vi "Chat Message Callback.vi"(7 "Owner":refnum<class>, 11 "Message":refnum<class "Message.lvclass">) -> (0 "error out":errorcluster)   [LabVIEW 2020, in "LV Chat Server.lvclass"]
uses:
  LV Chat Server.lvclass
  <vilib>/IlluminatedG/lv-msg-simple/Stream-Simple-Msg/Message/Message.lvclass
  LV Chat Server.lvclass/LV Chat Server.ctl
  Data Types/Message.ctl
  Data Types/Message ID.ctl
  9b2631c7-d2a0-400d-8d9b-28026d0b08d4.vi
  8fd8f42d-e5b1-4272-a4de-ff1efb915e34.vi
  a0ad2d85-71bd-4b38-8ce3-2817e254df22.vi
  a0ad2d85-71bd-4b38-8ce3-2817e254df22.vi/43e93f4b-eb60-4448-b7e4-56a49cc750fb.vi
  a0ad2d85-71bd-4b38-8ce3-2817e254df22.vi/43e93f4b-eb60-4448-b7e4-56a49cc750fb.vi/4b61994f-5270-44fc-a580-5e93e6c23fba.vi
  <vilib>/IlluminatedG/lv-stream/stream/Write Formatted Data.vi
  <vilib>/IlluminatedG/lv-msg-simple/Stream-Simple-Msg/Message/Data and Type.vi
  <vilib>/IlluminatedG/lv-msg-simple/Stream-Simple-Msg/Manager/Get Endpoints.vi
  <vilib>/IlluminatedG/lv-msg-simple/Stream-Simple-Msg/Endpoint/Get Stream.vi
  <vilib>/IlluminatedG/lv-stream/stream/Get Mode.vi
  <vilib>/IlluminatedG/lv-stream/stream/Prepared.vi
  <vilib>/Utility/error.llb/Error Cluster From Error Code.vi
  <vilib>/IlluminatedG/lv-stream/stream/Dispatch Sniffer Data.vi
  <vilib>/IlluminatedG/lv-stream/stream/Stream.lvclass
  <vilib>/IlluminatedG/lv-msg-simple/Stream-Simple-Msg/Endpoint/Endpoint.lvclass
  <vilib>/IlluminatedG/lv-stream/URI/URI.lvclass
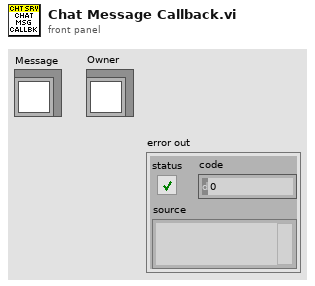
[diagram p1: front panel]
types:
  T1 = typedef "LV Chat Server.lvclass/Ref Data.ctl" = cluster{"Endpoint Map":map{string, T2}, "User Map":map{string, string}}
  T2 = typedef "LV Chat Server.lvclass/User.ctl" = cluster{"Name":string, "IP":string, "Connected At":dbl, "Endpoint":refnum<class "Endpoint.lvclass">}
  T3 = typedef "Message ID.ctl" = enum16{"UserInfo", "UserList", "Message", "Disconnect"}
  T4 = typedef "Message.ctl" = cluster{"From":string, "Time":dbl, "Message":string}
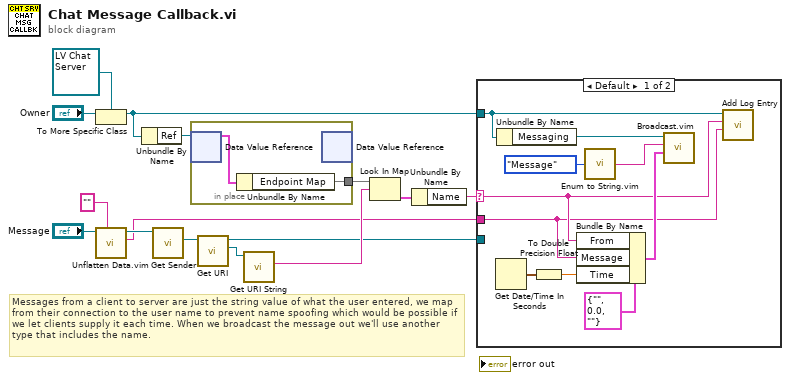
[diagram p0: block diagram]
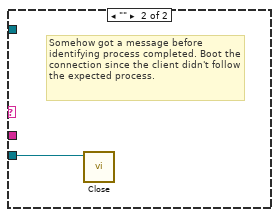
[diagram p2: hidden frame]
diagram:
  # "Messages from a client to server are just the string value of what the user entered, we map from their connection to the user name to prevent name spoofing which would be possible if we let clients supply it each time. When we broadcast the message out we'll use another type that includes the name."
  n1 = To More Specific Class(target class=refnum<class "LV Chat Server.lvclass"> refnum ("LV Chat Server.lvclass"), reference="Owner") -> (specific class reference=w1:refnum<class "LV Chat Server.lvclass">)  [unwired: 1 in, 1 out]
  n2 = call "Unflatten Data.vim"("Data Type (String)"="", "Message in"="Message") -> ("Unflattened Data"=w3:string, "Message out"=w11:refnum<class "Message.lvclass">)  [unwired: 7 in, 1 out]
  n3 = Unbundle By Name(w1) -> ("Ref"=w8:refnum<data-value>)
  n4 = call <vilib>:"Get Sender.vi"("Message in"=w11) -> ("Sender"=w10:refnum<class "Endpoint.lvclass">)  [unwired: 8 in, 2 out]
  n5 = in-place {
    in-place-border: [w16] -> w7
    n6 = in-place-dvr #1(w8) -> (w17:T1)  [unwired: 1 out]
    n7 = Unbundle By Name(w17) -> ("Endpoint Map"=w16:map{string, T2})
    n8 = in-place-dvr #1() -> ()  [unwired: 1 in, 2 out]
  }
  n9 = call <vilib>:"Get URI.vi"("Endpoint in"=w10) -> ("URI"=w9:refnum<class "URI.lvclass">, "Endpoint out"=w2:refnum<class "Endpoint.lvclass">)  [unwired: 8 in, 1 out]
  n10 = call <vilib>:"Get URI String.vi"("URI in"=w9) -> ("URI String"=w6:string)  [unwired: 8 in, 2 out]
  n11 = Look In Map(map=w7, key=w6) -> (value=w5:T2)  [unwired: 1 in, 1 out]
  n12 = Unbundle By Name(w5) -> ("Name"=w4:string)
  n13 = case shown="Default" w4 {
    selector: w4 -> [w19 _]
    tunnel: w3 -> [w18 _]
    tunnel: w2 -> [_ w28]
    tunnel: w1 -> [w20 _]
    frame Default {
      n14 = Get Date/Time In Seconds() -> (seconds since 1Jan1904=w26:timestamp)
      n15 = Unbundle By Name(w20) -> ("Messaging"=w24:refnum<class "Manager.lvclass">)
      n16 = To Double Precision Float(number=w26) -> (double precision float=w25:dbl)
      n17 = Bundle By Name(cluster=T4 {"From"="", "Time"=0.0, "Message"=""} ("Message"), "From"=w19, "Message"=w18, "Time"=w25) -> (w23:T4)
      n18 = call "Enum to String.vim"("Enum"=Message_ID."Message" ("Message ID")) -> ("Enum String"=w21:string)
      n19 = call "Broadcast.vim"("Data"=w23, "ID"=w21, "Manager in"=w24) -> ()  [unwired: 7 in, 2 out]
      n20 = call "Add Log Entry.vi"("Message"=w18, "From (SERVER)"=w19, "LV Chat Server in"=w20) -> ()  [unwired: 7 in, 2 out]
    }
    frame "" {
      # "Somehow got a message before identifying process completed. Boot the connection since the client didn't follow the expected process."
      n21 = call <vilib>:"Close.vi"("Endpoint in"=w28) -> ()  [unwired: 10 in, 1 out]
    }
  }
